vi "EnterEnglishWord.vi"(2 "?":bool, 8 "error in (no error)":errorcluster, 11 "Enter Translation In English":string) -> (0 "error out":errorcluster, 1 "Cancelled":bool, 3 "English":string)   [LabVIEW 2020]
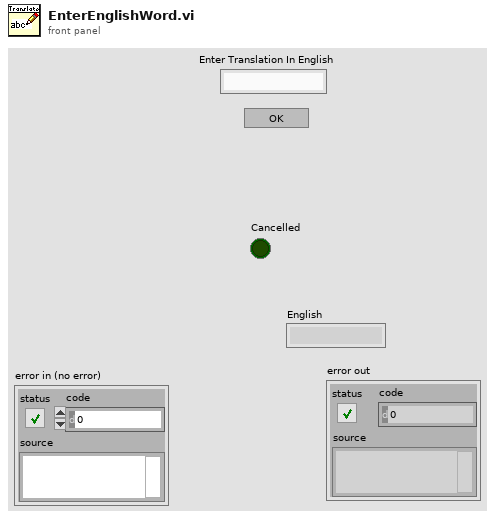
[diagram p1: front panel]
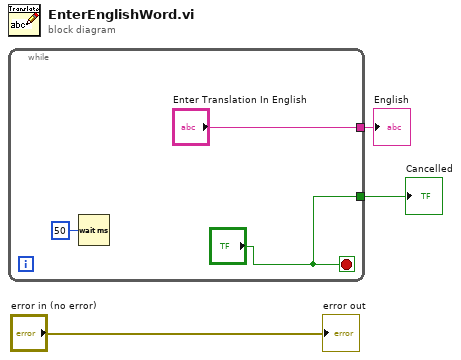
[diagram p0: block diagram]
diagram:
  n1 = while {
    tunnel: ["Enter Translation In English"] -> w2
    tunnel: ["?"] -> w1
    stop <- "?" stop-if-true
    n2 = Wait (ms)(milliseconds to wait=u32 50) -> ()  [unwired: 1 out]
  }
  "English" <- w2
  "Cancelled" <- w1
  "error out" <- "error in (no error)"
